vi "Deadzone.vi"(3 "Default":dbl, 4 "Array(in)":dbl[](array[numeric]), 5 "Deadzone":dbl) -> (1 "Array(out)":dbl[](array[numeric]))   [LabVIEW 2012]
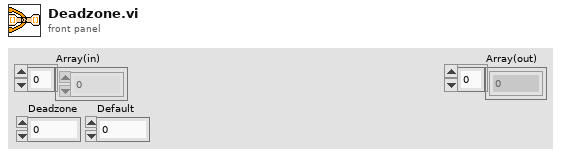
[diagram p1: front panel]
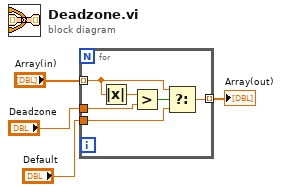
[diagram p0: block diagram]
diagram:
  n1 = for {
    tunnel: "Array(in)" -> [w8] mode=indexing
    tunnel: "Deadzone" -> [w7]
    tunnel: [w6] -> w2 mode=indexing
    tunnel: "Default" -> [w5]
    n2 = Absolute Value(x=w8) -> (abs(x)=w9:dbl)
    n3 = Greater?(x=w9, y=w7) -> (0:w10:bool)
    n4 = Select(t=w8, s=w10, f=w5) -> (s? t:f=w6:dbl)
  }
  "Array(out)" <- w2
